vi "sec_div_selector.vi"(2 "error in (no error)":errorcluster, 3 "Esponente":enum16{"ns", "us", "ms", "s"}(ring), 4 "Sec a divisione":enum16{"1", "2,5", "5"}(ring)) -> (0 "error out":errorcluster, 1 "sec/div":ext)   [LabVIEW 2022 SP3]
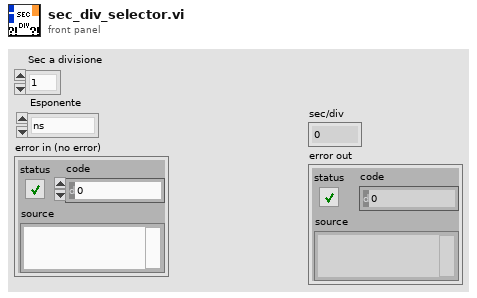
[diagram p1: front panel]
types:
  T1 = cluster{"status":bool, "code":i32, "error source (\" \")":string}
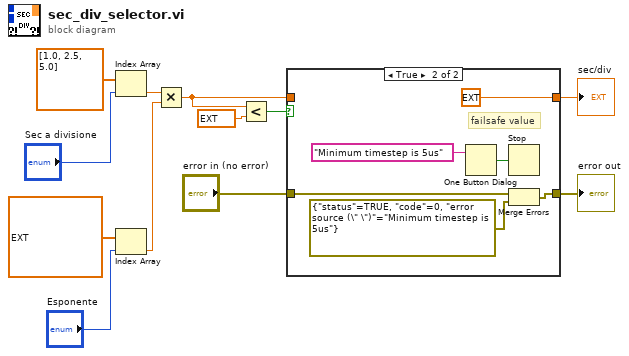
[diagram p0: block diagram]
diagram:
  n1 = Index Array(array=sgl[] [1.0, 2.5, 5.0], index="Sec a divisione") -> (element=w7:sgl)
  n2 = Index Array(array=ext[] [1e-9, 0.00000100000000000000000004, 0.00099999999999999999996, 1.0, 0.0, 0.0], index="Esponente") -> (element=w8:ext)
  n3 = Multiply(x=w7, y=w8) -> (x*y=w2:ext)
  n4 = Less?(x=w2, y=ext 4.9e-9) -> (x < y?=w5:bool)
  n5 = case shown="True" w5 {
    tunnel: [w14 w19] -> w4
    tunnel: "error in (no error)" -> [w14 w20]
    tunnel: w2 -> [w13 _]
    tunnel: [w13 ext 1.0] -> w1
    frame False {
    }
    frame True {
      # "failsafe value"
      n6 = One Button Dialog(message="Minimum timestep is 5us" ("error source (\" \")")) -> (true=w17:bool)  [unwired: 1 in]
      n7 = Stop(stop? (T)=w17) -> ()
      n8 = Merge Errors(w20, T1 {"status"=TRUE, "code"=0, "error source (\" \")"="Minimum timestep is 5us"} ("error constant")) -> (w19:errorcluster)
    }
  }
  "error out" <- w4
  "sec/div" <- w1
